vi "Write Test Group Database.vi"(8 "error in (no error)":errorcluster, 10 "Test Group Database":variant, 11 "Test Group Manager in":refnum<class "Test Group Manager.lvclass">) -> (0 "error out":errorcluster, 3 "Test Group Manager out":refnum<class "Test Group Manager.lvclass">)   [LabVIEW 2016, in "Test Group Manager.lvlib" / "Test Group Manager.lvclass"]
uses:
  Test Group Manager.lvclass
  Test Group Manager.lvclass/Test Group Manager.ctl
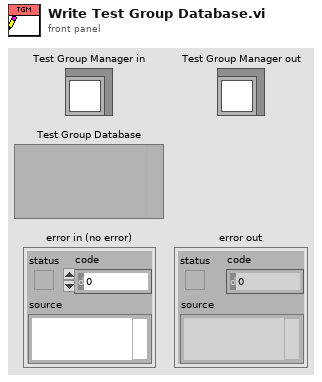
[diagram p1: front panel]
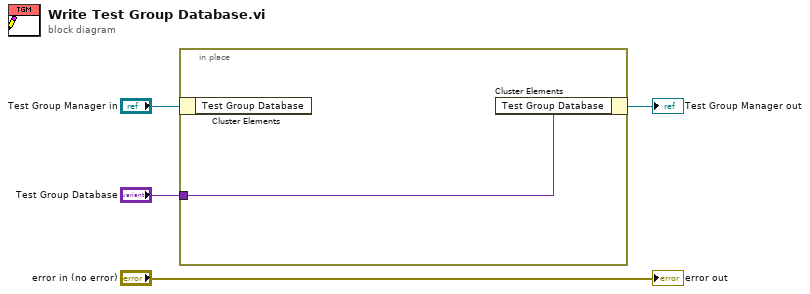
[diagram p0: block diagram]
diagram:
  n1 = in-place {
    in-place-border: "Test Group Database" -> [w5]
    n2 = in-place-cluster #1("Test Group Manager in") -> ()  [unwired: 1 out]
    n3 = in-place-cluster #1("Test Group Database"=w5) -> (→"Test Group Manager out":refnum<class "Test Group Manager.lvclass">)
  }
  "error out" <- "error in (no error)"
